vi "Finish.vi"   [LabVIEW 2013]
doc: "This VI is called just before exiting. It is expected to close I/O refnum, save collected data, etc."
uses:
  <vilib>/Rock Robotics/WPI/Relay/WPI_RelayValue.ctl
  <vilib>/Rock Robotics/WPI/Compressor/WPI_CompressorGetSetRefNum.vi
  <vilib>/Rock Robotics/WPI/Joystick/WPI_JoystickGetSetRefNum.vi
  <vilib>/Rock Robotics/WPI/RobotDrive/WPI_RobotDriveGetSetRefNum.vi
types:
  T1 = typedef "WPI_RelayValue.ctl" = enum16{"Off", "On", "Forward", "Reverse"}
  T2 = typedef "WPI_JoystickDevRef.ctl" = cluster{"Device":T3}
  T3 = typedef "WPI_JoystickDeviceEnum.ctl" = enum16{"USB 1", "USB 2", "USB 3", "USB 4", "Kinect 1", "Kinect 2"}
  T4 = typedef "WPI_RobotDriveDevRef.ctl" = cluster{"DevStatus":errorcluster, "Motors[]":T5[], "Square Inputs":bool, "Max Output":dbl, "Isochronous":bool}
  T5 = typedef "WPI_MotorControlDeviceRef.ctl" = cluster{"DeviceStatus":errorcluster, "Type":enum16{"PWM", "CAN"}, "PWM":cluster{"Digital Module":T6, "PWM Channel":T7, "DeadBand":T8}, "CAN":cluster{"Device Number":u8, "Control Mode":T9, "Semaphore":T10, "Max Vout":dbl}, "Invert":bool, "TransformRef":T11, "InvTransformRef":T11}
  T6 = typedef "FPGA_TypedefDigitalModule.ctl" = enum16{"Digital Module 1", "Digital Module 2"}
  T7 = typedef "FPGA_DIOPWMChannel.ctl" = enum8{"PWM 1", "PWM 2", "PWM 3", "PWM 4", "PWM 5", "PWM 6", "PWM 7", "PWM 8", "PWM 9", "PWM 10", "Invalid"}
  T8 = typedef "WPI_PWMDeadband.ctl" = cluster{"Name":string, "maxPositivePwm":i32, "minPositivePwm":i32, "centerPwm":i32, "maxNegativePwm":i32, "minNegativePwm":i32, "angularRange":u16}
  T9 = typedef "WPI_CANJaguar_ControlMode.ctl" = enum8{"Percent VBus", "Current", "Speed", "Position", "Voltage"}
  T10 = typedef "Semaphore RefNum" = refnum<k1>
  T11 = typedef "WPI_PWMTransform_ConPane.ctl" = refnum<vi>
  T12 = typedef "WPI_AnalogChannelDevRef.ctl" = cluster{"DevStatus":errorcluster, "Analog Module":T13, "Analog Channel":T14}
  T13 = typedef "FPGA_TypedefAnalogModule.ctl" = enum16{"Analog Module 1", "Analog Module 2"}
  T14 = typedef "FPGA_AIChannel.ctl" = enum8{"AI 1", "AI 2", "AI 3", "AI 4", "AI 5", "AI 6", "AI 7", "AI 8", "Invalid"}
  T15 = typedef "WPI_EncoderDevRef.ctl" = cluster{"DevStatus":errorcluster, "EncoderIndex":T16, "CounterIndex":T17, "DistancePerCount":dbl, "Decoding Type":T18}
  T16 = typedef "FPGA_EncoderIdx.ctl" = enum8{"Enc 0", "Enc 1", "Enc 2", "Enc 3", "Invalid"}
  T17 = typedef "FPGA_CounterCtrSystemIndex.ctl" = enum8{"Ctr 0", "Ctr 1", "Ctr 2", "Ctr 3", "Ctr 4", "Ctr 5", "Ctr 6", "Ctr 7", "Invalid"}
  T18 = typedef "WPI_EncoderType.ctl" = enum16{"1x", "2x", "4x"}
  T19 = typedef "WPI_SolenoidDevRef.ctl" = cluster{"DevStatus":errorcluster, "Solenoid Module":T20, "Forward Solenoid Channel":T21, "Reverse Solenoid Channel":T21}
  T20 = typedef "FPGA_TypedefSolenoidModule.ctl" = enum16{"Solenoid Module 1", "Solenoid Module 2"}
  T21 = typedef "WPI_SolenoidChannel.ctl" = enum8{"Solenoid 1", "Solenoid 2", "Solenoid 3", "Solenoid 4", "Solenoid 5", "Solenoid 6", "Solenoid 7", "Solenoid 8", "Invalid"}
  T22 = typedef "WPI_CompressorDevRef.ctl" = cluster{"DevStatus":errorcluster, "DigitalInputDevRef":T23, "RelayDevRef":T25}
  T23 = typedef "WPI_DigitalInputDevRef.ctl" = cluster{"DevStatus":errorcluster, "DIO Channel":T24, "Digital Module":T6}
  T24 = typedef "FPGA_DIOChannel.ctl" = enum8{"DIO 1", "DIO 2", "DIO 3", "DIO 4", "DIO 5", "DIO 6", "DIO 7", "DIO 8", "DIO 9", "DIO 10", "DIO 11", "DIO 12", "DIO 13", "DIO 14", "Invalid"}
  T25 = typedef "WPI_RelayDevRef.ctl" = cluster{"DevStatus":errorcluster, "Relay Channel":T26, "Digital Module":T6, "Relay Direction":T27}
  T26 = typedef "FPGA_DIORelayChannel.ctl" = enum8{"Relay 1", "Relay 2", "Relay 3", "Relay 4", "Relay 5", "Relay 6", "Relay 7", "Relay 8", "Invalid"}
  T27 = typedef "WPI_RelayDirection.ctl" = enum16{"Both directions", "Forward only", "Reverse only"}
  T28 = typedef "WPI_GyroDevRef.ctl" = cluster{"DevStatus":errorcluster, "Analog Module":T13, "Analog Channel":T14, "Offset":dbl, "Gain (VoltsPerDegree/Second)":dbl}
  T29 = typedef "WPI_DigitalOutputDevRef.ctl" = cluster{"Digital Module":T6, "DIO Channel":T24, "DevStatus":errorcluster}
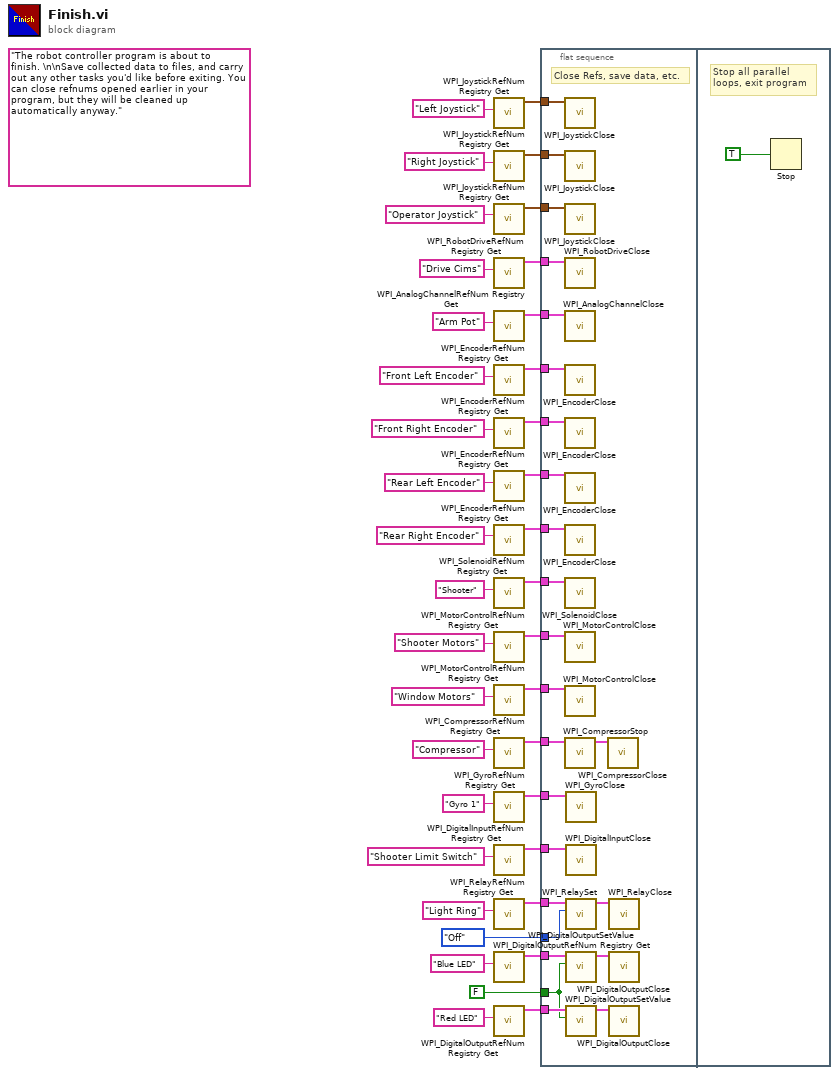
[diagram p0: block diagram]
diagram:
  (unwired) "The robot controller program is about to finish. \n\nSave collected data to files, and carry out any other tasks you'd like before exiting. You can close refnums opened earlier in your program, but they will be cleaned up automatically anyway."
  n1 = call <vilib>:"WPI_JoystickRefNum Registry Get.vi"("refnum name"="Left Joystick") -> ("JoystickDevRef"=w35:T2)  [unwired: 1 in, 9 out]
  n2 = call <vilib>:"WPI_JoystickRefNum Registry Get.vi"("refnum name"="Right Joystick") -> ("JoystickDevRef"=w33:T2)  [unwired: 1 in, 9 out]
  n3 = call <vilib>:"WPI_JoystickRefNum Registry Get.vi"("refnum name"="Operator Joystick") -> ("JoystickDevRef"=w32:T2)  [unwired: 1 in, 9 out]
  n4 = call <vilib>:"WPI_RobotDriveRefNum Registry Get.vi"("refnum name"="Drive Cims") -> ("RobotDriveDevRef"=w36:T4)  [unwired: 1 in, 9 out]
  n5 = call <vilib>:"WPI_AnalogChannelRefNum Registry Get.vi"("refnum name"="Arm Pot") -> ("AIDeviceRef"=w30:T12)  [unwired: 9 in, 1 out]
  n6 = call <vilib>:"WPI_EncoderRefNum Registry Get.vi"("refnum name"="Front Left Encoder") -> ("EncoderDevRef"=w28:T15)  [unwired: 9 in, 1 out]
  n7 = call <vilib>:"WPI_EncoderRefNum Registry Get.vi"("refnum name"="Front Right Encoder") -> ("EncoderDevRef"=w25:T15)  [unwired: 9 in, 1 out]
  n8 = call <vilib>:"WPI_EncoderRefNum Registry Get.vi"("refnum name"="Rear Left Encoder") -> ("EncoderDevRef"=w10:T15)  [unwired: 9 in, 1 out]
  n9 = call <vilib>:"WPI_EncoderRefNum Registry Get.vi"("refnum name"="Rear Right Encoder") -> ("EncoderDevRef"=w9:T15)  [unwired: 9 in, 1 out]
  n10 = call <vilib>:"WPI_SolenoidRefNum Registry Get.vi"("refnum name"="Shooter") -> ("SolenoidDevRef"=w23:T19)  [unwired: 9 in, 1 out]
  n11 = call <vilib>:"WPI_MotorControlRefNum Registry Get.vi"("refnum name"="Shooter Motors") -> ("MotorControlDevRef"=w22:T5)  [unwired: 9 in, 1 out]
  n12 = call <vilib>:"WPI_MotorControlRefNum Registry Get.vi"("refnum name"="Window Motors") -> ("MotorControlDevRef"=w15:T5)  [unwired: 9 in, 1 out]
  n13 = call <vilib>:"WPI_CompressorRefNum Registry Get.vi"("refnum name"="Compressor") -> ("CompressorDevRef"=w20:T22)  [unwired: 9 in, 1 out]
  n14 = call <vilib>:"WPI_GyroRefNum Registry Get.vi"("refnum name"="Gyro 1") -> ("GyroDevRef"=w18:T28)  [unwired: 9 in, 1 out]
  n15 = call <vilib>:"WPI_DigitalInputRefNum Registry Get.vi"("refnum name"="Shooter Limit Switch") -> ("DigitalInputDevRef"=w14:T23)  [unwired: 9 in, 1 out]
  n16 = call <vilib>:"WPI_RelayRefNum Registry Get.vi"("refnum name"="Light Ring") -> ("RelayDevRef"=w4:T25)  [unwired: 9 in, 1 out]
  n17 = call <vilib>:"WPI_DigitalOutputRefNum Registry Get.vi"("refnum name"="Blue LED") -> ("DigitalOutputDevRef"=w7:T29)  [unwired: 9 in, 1 out]
  n18 = call <vilib>:"WPI_DigitalOutputRefNum Registry Get.vi"("refnum name"="Red LED") -> ("DigitalOutputDevRef"=w5:T29)  [unwired: 9 in, 1 out]
  n19 = flat-sequence {
    tunnel: w36 -> [w62]
    tunnel: w35 -> [w61]
    tunnel: w33 -> [w60]
    tunnel: w32 -> [w59]
    tunnel: w30 -> [w58]
    tunnel: w28 -> [w50]
    tunnel: w25 -> [w49]
    tunnel: w23 -> [w57]
    tunnel: w22 -> [w56]
    tunnel: w20 -> [w54]
    tunnel: w18 -> [w53]
    tunnel: w15 -> [w52]
    tunnel: w14 -> [w51]
    tunnel: w10 -> [w48]
    tunnel: w9 -> [w47]
    tunnel: w7 -> [w46]
    tunnel: w5 -> [w45]
    tunnel: w4 -> [w42]
    tunnel: WPI_RelayValue."Off" ("RelayValue") -> [w41]
    tunnel: FALSE ("Value") -> [w39]
    frame #0 {
      # "Close Refs, save data, etc."
      n20 = call <vilib>:"WPI_JoystickClose.vi"("JoystickDevRef"=w61) -> ()  [unwired: 11 out]
      n21 = call <vilib>:"WPI_JoystickClose.vi"("JoystickDevRef"=w60) -> ()  [unwired: 11 out]
      n22 = call <vilib>:"WPI_JoystickClose.vi"("JoystickDevRef"=w59) -> ()  [unwired: 11 out]
      n23 = call <vilib>:"WPI_RobotDriveClose.vi"("RobotDriveDevRef"=w62) -> ()  [unwired: 1 in, 10 out]
      n24 = call <vilib>:"WPI_AnalogChannelClose.vi"("AIDeviceRef"=w58) -> ()  [unwired: 10 in, 1 out]
      n25 = call <vilib>:"WPI_EncoderClose.vi"("EncoderDevRef"=w50) -> ()  [unwired: 10 in, 1 out]
      n26 = call <vilib>:"WPI_EncoderClose.vi"("EncoderDevRef"=w49) -> ()  [unwired: 10 in, 1 out]
      n27 = call <vilib>:"WPI_EncoderClose.vi"("EncoderDevRef"=w48) -> ()  [unwired: 10 in, 1 out]
      n28 = call <vilib>:"WPI_EncoderClose.vi"("EncoderDevRef"=w47) -> ()  [unwired: 10 in, 1 out]
      n29 = call <vilib>:"WPI_SolenoidClose.vi"("SolenoidDevRef"=w57) -> ()  [unwired: 10 in, 1 out]
      n30 = call <vilib>:"WPI_MotorControlClose.vi"("MotorControlDevRef"=w56) -> ()  [unwired: 10 in, 1 out]
      n31 = call <vilib>:"WPI_MotorControlClose.vi"("MotorControlDevRef"=w52) -> ()  [unwired: 10 in, 1 out]
      n32 = call <vilib>:"WPI_CompressorStop.vi"("CompressorDevRef"=w54) -> ("CompressorDevRef"=w55:T22)  [unwired: 9 in, 1 out]
      n33 = call <vilib>:"WPI_GyroClose.vi"("GyroDevRef"=w53) -> ()  [unwired: 10 in, 1 out]
      n34 = call <vilib>:"WPI_DigitalInputClose.vi"("DigitalInputDevRef"=w51) -> ()  [unwired: 10 in, 1 out]
      n35 = call <vilib>:"WPI_RelaySet.vi"("RelayValue"=w41, "RelayDevRef"=w42) -> ("RelayDevRef"=w40:T25)  [unwired: 8 in, 1 out]
      n36 = call <vilib>:"WPI_DigitalOutputSetValue.vi"("Value"=w39, "DigitalOutputDevRef"=w46) -> ("DigitalOutputDevRef"=w44:T29)  [unwired: 8 in, 1 out]
      n37 = call <vilib>:"WPI_DigitalOutputSetValue.vi"("Value"=w39, "DigitalOutputDevRef"=w45) -> ("DigitalOutputDevRef"=w43:T29)  [unwired: 8 in, 1 out]
      n38 = call <vilib>:"WPI_CompressorClose.vi"("CompressorDevRef"=w55) -> ()  [unwired: 10 in, 1 out]
      n39 = call <vilib>:"WPI_RelayClose.vi"("RelayDevRef"=w40) -> ()  [unwired: 10 in, 1 out]
      n40 = call <vilib>:"WPI_DigitalOutputClose.vi"("DigitalOutputDevRef"=w44) -> ()  [unwired: 10 in, 1 out]
      n41 = call <vilib>:"WPI_DigitalOutputClose.vi"("DigitalOutputDevRef"=w43) -> ()  [unwired: 10 in, 1 out]
    }
    frame #1 {
      # "Stop all parallel\nloops, exit program"
      n42 = Stop(stop? (T)=TRUE ("Quit")) -> ()
    }
  }
